vi "Longer Pump dLSP501 Start Stop Run.vi"() -> ()   [LabVIEW 2023, in "Longer Pump dLSP501 Series.lvlib"]
uses:
  <instrlib>/Longer Pump dLSP501 Modbus RTU Series/Longer Pump dLSP501 Series.lvlib
  <vilib>/NI/Modbus Library/API/Master/Modbus Master.lvclass
  C:/Program Files/National Instruments/LabVIEW 2023/vi.lib/NI/Modbus Library/API/Modbus API.lvclass
  <instrlib>/Longer Pump dLSP501 Modbus RTU Series/Private/Initialize - Integrated Address.vi
panel:
  out "Error out":errorcluster caption="错误输出"
  in  "Error in":errorcluster caption="错误输入"
  in  "Open Port":bool caption="打开串口"
  in  "Stop Run":bool caption="停止"
  in  "Start Run":bool caption="启动"
  in  "Comm. Config.":T1={"Address"=1, "Baud Rate"=115200, "Parity"=0} caption="通讯设置" {"Parity" items=["无校验", "奇校验", "偶校验", "标记", "空格"]; "Baud Rate" items=["1200"=1200, "2400"=2400, "9600"=9600, "19200"=19200, "38400"=38400, "57600"=57600, "115200"=115200]}
  in  "VISA resource name":refnum<visa-resource-name>="COM1" caption="VISA资源名"
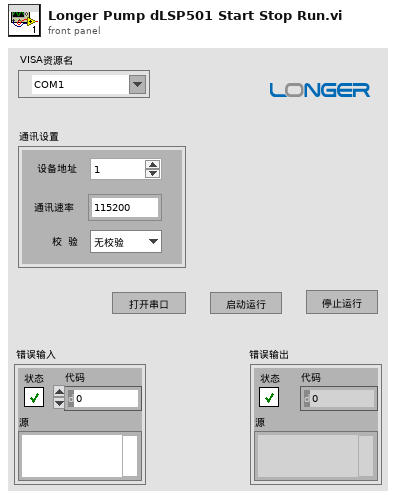
[diagram p1: front panel]
types:
  T1 = cluster{"Address":u8, "Baud Rate":u32, "Parity":u16}
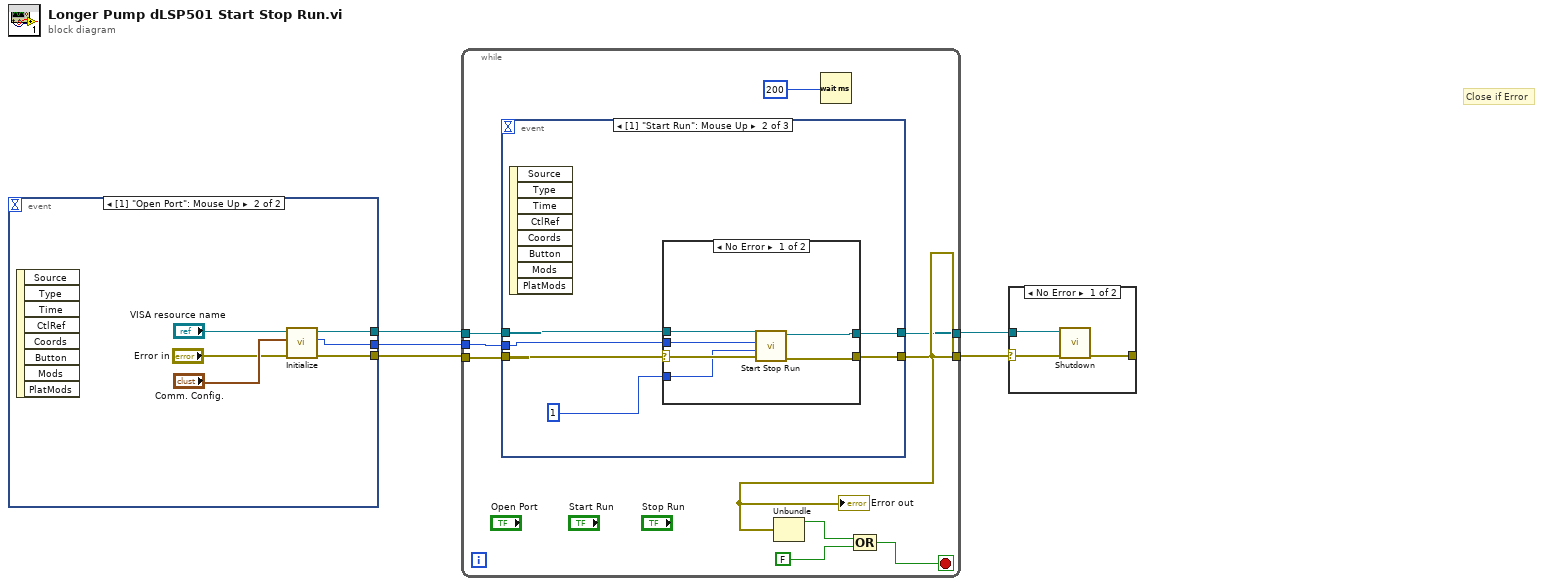
[diagram p0: block diagram]
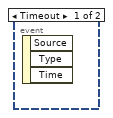
[diagram p2: hidden frame]
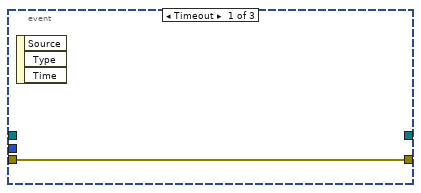
[diagram p4: hidden frame]
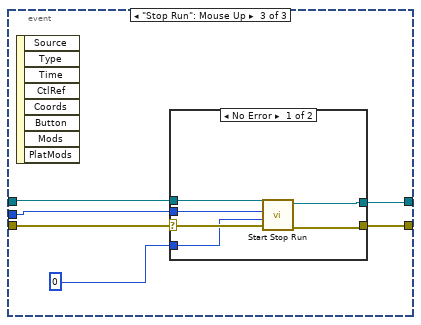
[diagram p6: hidden frame]
diagram:
  # "Close if Error"
  n1 = event shown="[1] \"Open Port\": Mouse Up" {
    selector: _ -> [_ _]
    dyn-events: _ -> [_ _]
    timeout: _ -> [_ _]
    tunnel: [_ w9] -> w3
    tunnel: [_ w8] -> w2
    tunnel: [_ w7] -> w1
    event Timeout {
      n2 = event-data() -> ()  [unwired: 1 in, 3 out]
    }
    event "Open Port": Mouse Up {
      n3 = event-data() -> ()  [unwired: 1 in, 8 out]
      n4 = call-poly <instrlib>:"Initialize.vi"("Error in"="Error in", "Comm. Config"="Comm. Config.", "VISA resource name"="VISA resource name") -> ("Error out"=w9:errorcluster, "Channel"=w8:i32, "serial master instance"=w7:refnum<class "Modbus Master.lvclass">)  [unwired: 5 in]
    }
  }
  n5 = while {
    tunnel: [w12] -> w5
    tunnel: [w15] -> w4
    tunnel: w3 -> [w17]
    tunnel: w1 -> [w16]
    tunnel: w2 -> [w13]
    stop <- w20 stop-if-true
    n6 = event shown="[1] \"Start Run\": Mouse Up" {
      selector: _ -> [_ _ _]
      dyn-events: _ -> [_ _ _]
      timeout: _ -> [_ _ _]
      tunnel: w17 -> [w21 w27 w41]
      tunnel: w16 -> [_ w26 w40]
      tunnel: [_ w25 w39] -> w15
      tunnel: [w21 w24 w38] -> w12
      tunnel: w13 -> [_ w23 w37]
      event Timeout {
        n7 = event-data() -> ()  [unwired: 1 in, 3 out]
      }
      event "Start Run": Mouse Up {
        n8 = event-data() -> ()  [unwired: 1 in, 8 out]
        n9 = case shown="No Error" w27 {
          selector: w27 -> [w32 w34]
          tunnel: w26 -> [w33 w35]
          tunnel: [w31 w35] -> w25
          tunnel: [w29 w34] -> w24
          tunnel: 1 -> [w30 _]
          tunnel: w23 -> [w28 _]
          frame No Error {
            n10 = call <instrlib>:"Start Stop Run.vi"("Error in"=w32, "Start/Stop"=w30, "Channel"=w28, "Modbus instance in"=w33) -> ("Error out"=w29:errorcluster, "Modbus instance out"=w31:refnum<class "Modbus Master.lvclass">)  [unwired: 6 in]
          }
          frame Error {
          }
        }
      }
      event "Stop Run": Mouse Up {
        n11 = event-data() -> ()  [unwired: 1 in, 8 out]
        n12 = case shown="No Error" w41 {
          selector: w41 -> [w46 w48]
          tunnel: w40 -> [w47 w49]
          tunnel: [w45 w49] -> w39
          tunnel: [w43 w48] -> w38
          tunnel: 0 -> [w44 _]
          tunnel: w37 -> [w42 _]
          frame No Error {
            n13 = call <instrlib>:"Start Stop Run.vi"("Error in"=w46, "Start/Stop"=w44, "Channel"=w42, "Modbus instance in"=w47) -> ("Error out"=w43:errorcluster, "Modbus instance out"=w45:refnum<class "Modbus Master.lvclass">)  [unwired: 6 in]
          }
          frame Error {
          }
        }
      }
    }
    "Error out" <- w12
    n14 = Unbundle(w12) -> ("status"=w18:bool)  [unwired: 2 out]
    n15 = Wait (ms)(milliseconds to wait=u32 200 ("毫秒计时值")) -> ()  [unwired: 1 out]
    n16 = Compound Arithmetic op=OR ("复合运算")(w18, FALSE ("Stop")) -> (w20:bool)
  }
  n17 = case shown="No Error" w5 {
    selector: w5 -> [w51 w53]
    tunnel: w4 -> [w52 _]
    tunnel: [w50 w53] -> _
    frame No Error {
      n18 = call-dynamic "Shutdown.vi"("error in"=w51, "Modbus master in"=w52) -> ("error out"=w50:errorcluster)  [unwired: 9 in]
    }
    frame Error {
    }
  }
